vi "Read Simulated Custom Devices.vi"(8 "error in (no error)":errorcluster, 11 "Simulated VeriStand Engine in":refnum<class "Simulated VeriStand Engine.lvclass">) -> (0 "error out":errorcluster, 2 "Simulated Custom Devices":refnum<class "Simulated VeriStand Custom Device.lvclass">[](array[class]), 3 "Simulated VeriStand Engine out":refnum<class "Simulated VeriStand Engine.lvclass">)   [LabVIEW 2016, in "Simulated VeriStand Engine.lvclass"]
uses:
  Simulated VeriStand Engine.lvclass
  Simulated VeriStand Custom Device/Simulated VeriStand Custom Device.lvclass
  Simulated VeriStand Engine.lvclass/Simulated VeriStand Engine.ctl
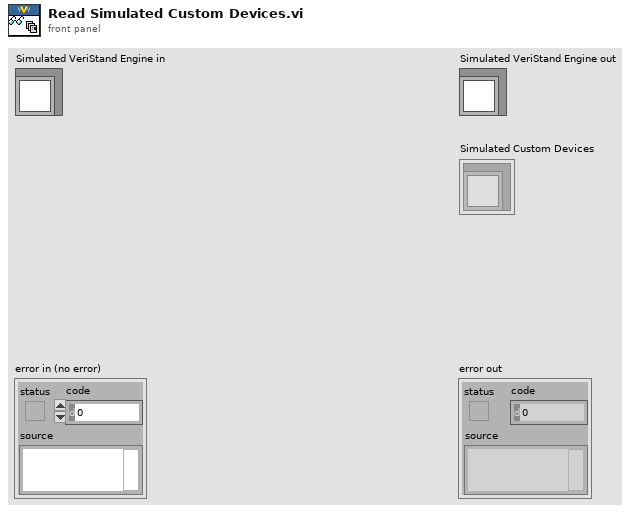
[diagram p1: front panel]
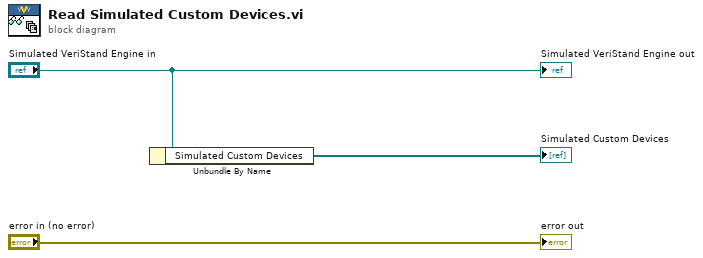
[diagram p0: block diagram]
diagram:
  n1 = Unbundle By Name("Simulated VeriStand Engine in") -> ("Simulated Custom Devices"=→"Simulated Custom Devices":refnum<class "Simulated VeriStand Custom Device.lvclass">[])
  "error out" <- "error in (no error)"
  "Simulated VeriStand Engine out" <- "Simulated VeriStand Engine in"
